vi "setup_furnitures.vi"(8 "error in":errorcluster, 11 "furntures in":refnum<class "IFurniture.lvclass">[](array[class])) -> (0 "error out":errorcluster, 1 "setup results":string[](array[string]), 3 "furntures out":refnum<class "IFurniture.lvclass">[](array[class]))   [LabVIEW 2021]
uses:
  IFurniture/IFurniture.lvclass
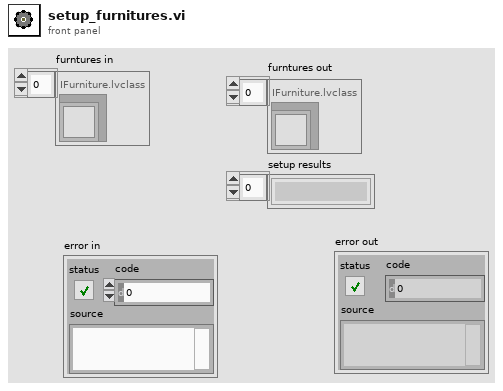
[diagram p1: front panel]
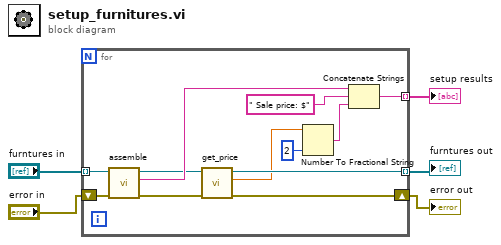
[diagram p0: block diagram]
diagram:
  n1 = for {
    tunnel: "furntures in" -> [w13] mode=indexing
    shift-right: [w7] -> w1
    shift-left: "error in" -> [w12]
    tunnel: [w9] -> w4 mode=indexing
    tunnel: [w14] -> w3 mode=indexing
    n2 = call-dynamic "assemble.vi"("error in (no error)"=w12, "IFurniture in"=w13) -> ("error out"=w6:errorcluster, "String"=w11:string, "IFurniture out"=w10:refnum<class "IFurniture.lvclass">)  [unwired: 7 in]
    n3 = call-dynamic "get_price.vi"("error in (no error)"=w6, "IFurniture in"=w10) -> ("error out"=w7:errorcluster, "price"=w8:dbl, "IFurniture out"=w9:refnum<class "IFurniture.lvclass">)  [unwired: 7 in]
    n4 = Number To Fractional String(number=w8, precision (6)=i16 2) -> (F-format string=w15:string)  [unwired: 2 in]
    n5 = Concatenate Strings(w11, " Sale price: $" ("string"), w15) -> (w14:string)
  }
  "furntures out" <- w4
  "setup results" <- w3
  "error out" <- w1
